vi "construct display.vi"(0 "input":T1(array[cluster]), 9 "Display in":string[][](array[string]), 11 "error in":errorcluster) -> (4 "Display out":string[][](array[string]), 6 "Highlighted lines":i32[](array[numeric]), 8 "Highlighted text":string[](array[string]), 10 "spreadsheet string":string, 13 "num cols":i32, 14 "num rows":i32, 15 "error out":errorcluster)   [LabVIEW 2018]
uses:
  <userlib>/_OpenG.lib/array/array.llb/Sort 1D Array (I32)__ogtk.vi
  <userlib>/_OpenG.lib/array/array.llb/Reorder 1D Array2 (String)__ogtk.vi
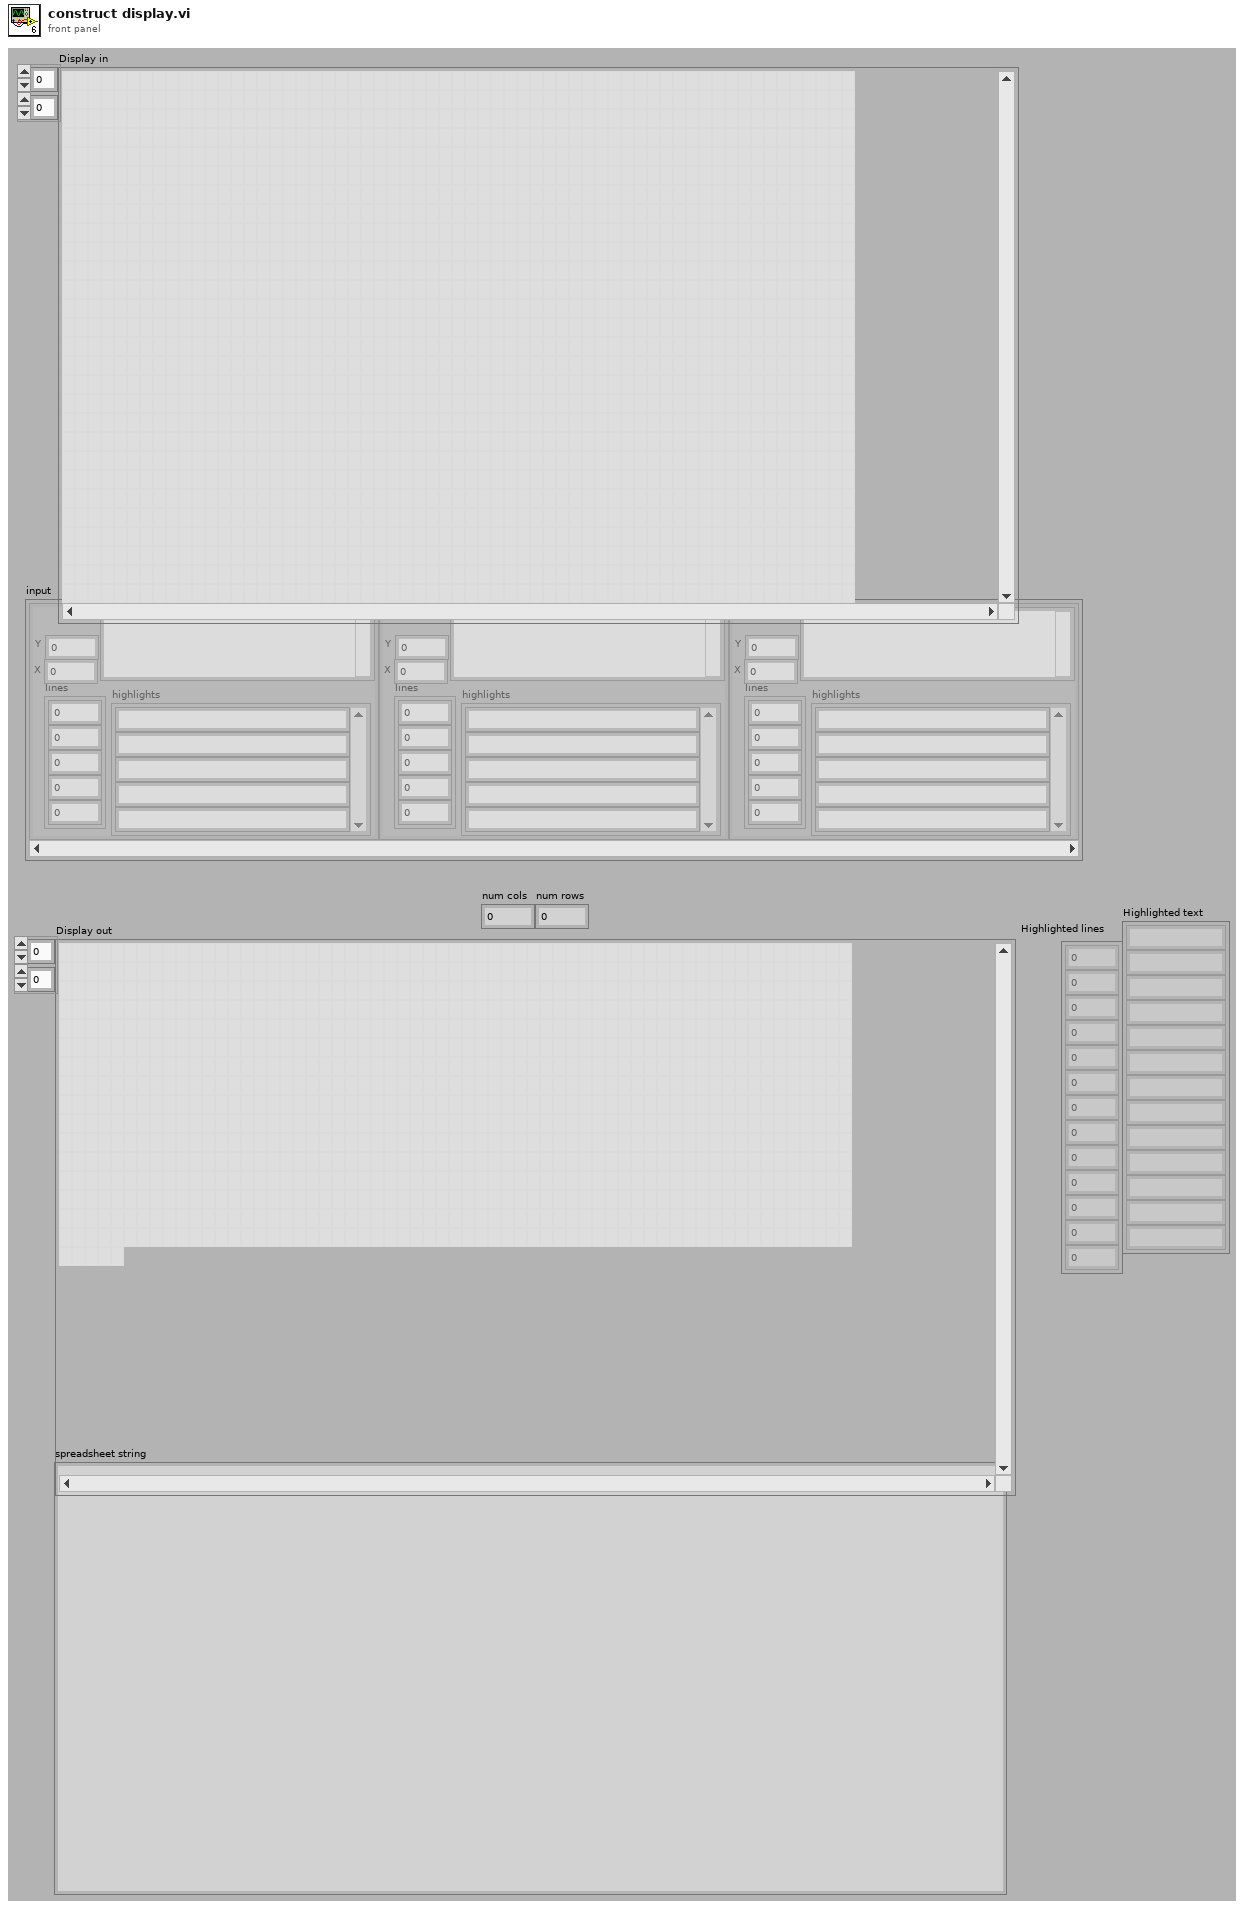
[diagram p1: front panel]
types:
  T1 = cluster{"Y":i32, "X":i32, "Text":string, "highlights":string[], "lines":i32[]}[]
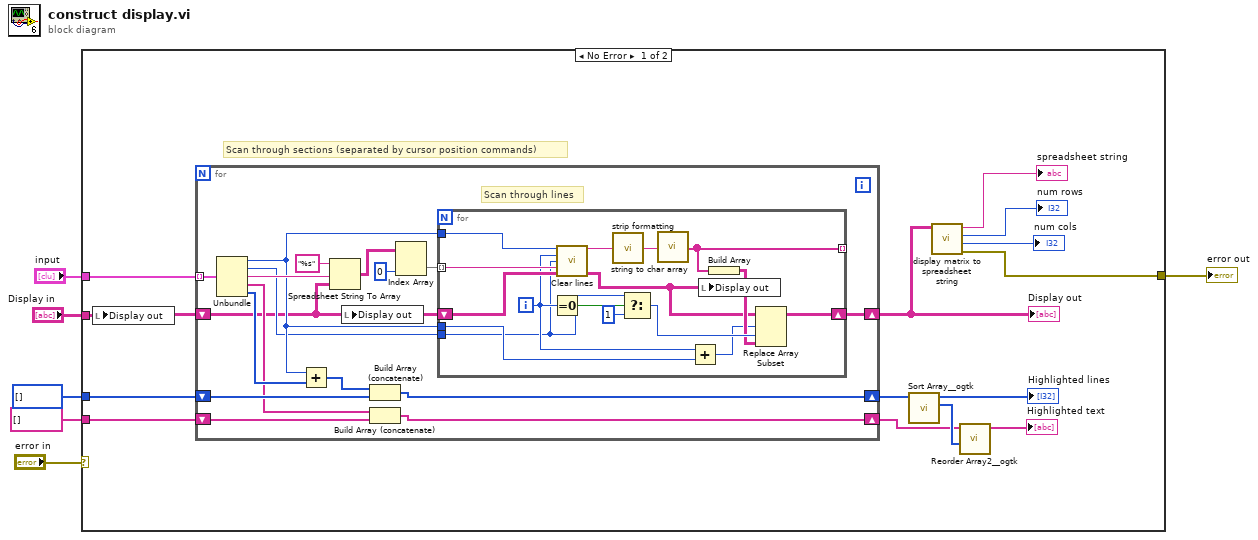
[diagram p0: block diagram]
diagram:
  n1 = case shown="No Error" "error in" {
    selector: "error in" -> [_ w54]
    tunnel: string[] [] -> [w15 _]
    tunnel: i32[] [] -> [w14 _]
    tunnel: "input" -> [w13 _]
    tunnel: "Display in" -> [w12 _]
    tunnel: [w7 w54] -> w2
    frame No Error {
      # "Scan through sections (separated by cursor position commands)"
      n2 = local write "Display out"(w12) -> ()
      n3 = for {
        tunnel: w13 -> [w36] mode=indexing
        shift-right: [w25] -> w11
        shift-left: w12 -> [w21]
        shift-right: [w29] -> w16
        shift-left: w14 -> [w30]
        shift-right: [w26] -> w18
        shift-left: w15 -> [w27]
        # "Scan through lines"
        n4 = Unbundle(w36) -> ("Y"=w24:i32, "X"=w23:i32, "Text"=w37:string, "highlights"=w28:string[], "lines"=w32:i32[])
        n5 = Add(x=w24, y=w32) -> (x+y=w31:i32[])
        n6 = Spreadsheet String To Array(format string="%s", spreadsheet string=w37, array type (2D Dbl)=w21) -> (array=w22:string[][])  [unwired: 1 in]
        n7 = local write "Display out"(w21) -> ()
        n8 = Build Array (concatenate)(w31, w30) -> (w29:i32[])
        n9 = Build Array (concatenate)(w28, w27) -> (w26:string[])
        n10 = Index Array(array=w22, index (col)=0 ("disabled index (col)")) -> (element=w34:string[])  [unwired: 1 in]
        n11 = for {
          tunnel: w34 -> [w53] mode=indexing
          tunnel: [w46] -> _ mode=indexing
          tunnel: w24 -> [w51]
          shift-right: [w45] -> w25
          shift-left: w21 -> [w52]
          tunnel: w24 -> [w43]
          tunnel: w23 -> [w38]
          i -> [w40]
          n12 = Equal To 0?(x=w40) -> (x = 0?=w41:bool)
          n13 = call "Clear lines.vi"("Section Y"=w51, "Section line"=w40, "Section X"=w38, "Section text"=w53, "Display Array"=w52) -> ("Stripped text"=w50:string, "Cleared Display Array"=w39:string[][])  [unwired: 9 in]
          n14 = call "strip formatting.vi"("result string 2"=w50) -> ("result string"=w49:string)
          n15 = Select(t=w38, s=w41, f=1) -> (s? t:f=w48:i32)
          n16 = call "string to char array.vi"("Stripped text"=w49) -> ("Array"=w46:string[])
          n17 = Add(x=w40, y=w43) -> (x+y=w42:i32)
          n18 = local write "Display out"(w39) -> ()
          n19 = Build Array(w46) -> (w44:string[][])
          n20 = Replace Array Subset(array=w39, new element=w44, index (row)=w42, index (col)=w48) -> (w45:string[][])
        }
      }
      "Display out" <- w11
      n21 = call-poly <userlib>:"Sort Array__ogtk.vi"("Array in"=w16) -> ("Sorted Pointers"=w19:i32[], "Sorted Array out"=→"Highlighted lines":i32[])  [unwired: 9 in]
      n22 = call "display matrix to spreadsheet string.vi"("Display"=w11) -> ("error out"=w7:errorcluster, "num cols"=→"num cols":i32, "num rows"=→"num rows":i32, "spreadsheet string"=→"spreadsheet string":string)  [unwired: 7 in]
      n23 = call-poly <userlib>:"Reorder Array2__ogtk.vi"("indices"=w19, "array"=w18) -> ("reordered array"=→"Highlighted text":string[])  [unwired: 9 in]
    }
    frame Error {
    }
  }
  "error out" <- w2
